vi "Read Setpoint Window.vi"(8 "error in (no error)":errorcluster, 11 "VISA resource name":refnum<visa-resource-name>) -> (0 "error out":errorcluster, 1 "Setpoint Window, C":dbl=2.0, 3 "VISA resource name out":refnum<visa-resource-name>)   [LabVIEW 2010, in "Temptronic TP04300.lvlib"]
doc: "This VI reads <b>Setpoint temperature window</b>\nValid Range: 0.1 to 9.9 \n\nNote: The window is the maximum positive or negative deviation from \nthe temperature setpoint allowable for an \"at temperature\" condition."
uses:
  Temptronic TP04300.lvlib
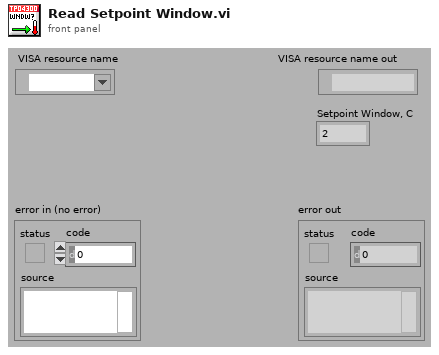
[diagram p1: front panel]
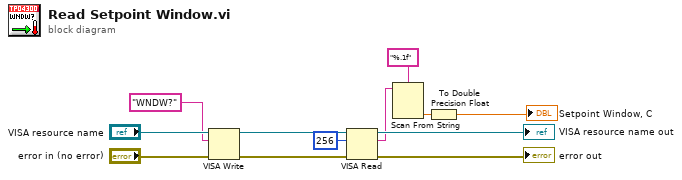
[diagram p0: block diagram]
diagram:
  n1 = VISA Write(VISA resource name="VISA resource name", write buffer="WNDW?" ("format string"), error in (no error)="error in (no error)") -> (VISA resource name out=w7:refnum<visa-resource-name>, error out=w10:errorcluster)  [unwired: 1 out]
  n2 = VISA Read(VISA resource name=w7, byte count=u32 256, error in (no error)=w10) -> (VISA resource name out=→"VISA resource name out":refnum<visa-resource-name>, read buffer=w5:string, error out=→"error out":errorcluster)  [unwired: 1 out]
  n3 = Scan From String(format string="%.1f", input string=w5) -> (output 1=w1:dbl)  [unwired: 3 in, 3 out]
  n4 = To Double Precision Float(number=w1) -> (double precision float=→"Setpoint Window, C":dbl)
